vi "robotmovingFinal.vi"() -> ()   [LabVIEW 2020]
uses:
  <vilib>/Instr/_visa.llb/VISA Configure Serial Port (Instr).vi
panel:
  out "read buffer":string
  in  "VISA resource name":refnum<visa-resource-name>="COM3"
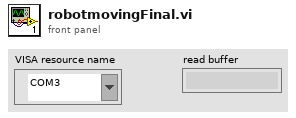
[diagram p1: front panel]
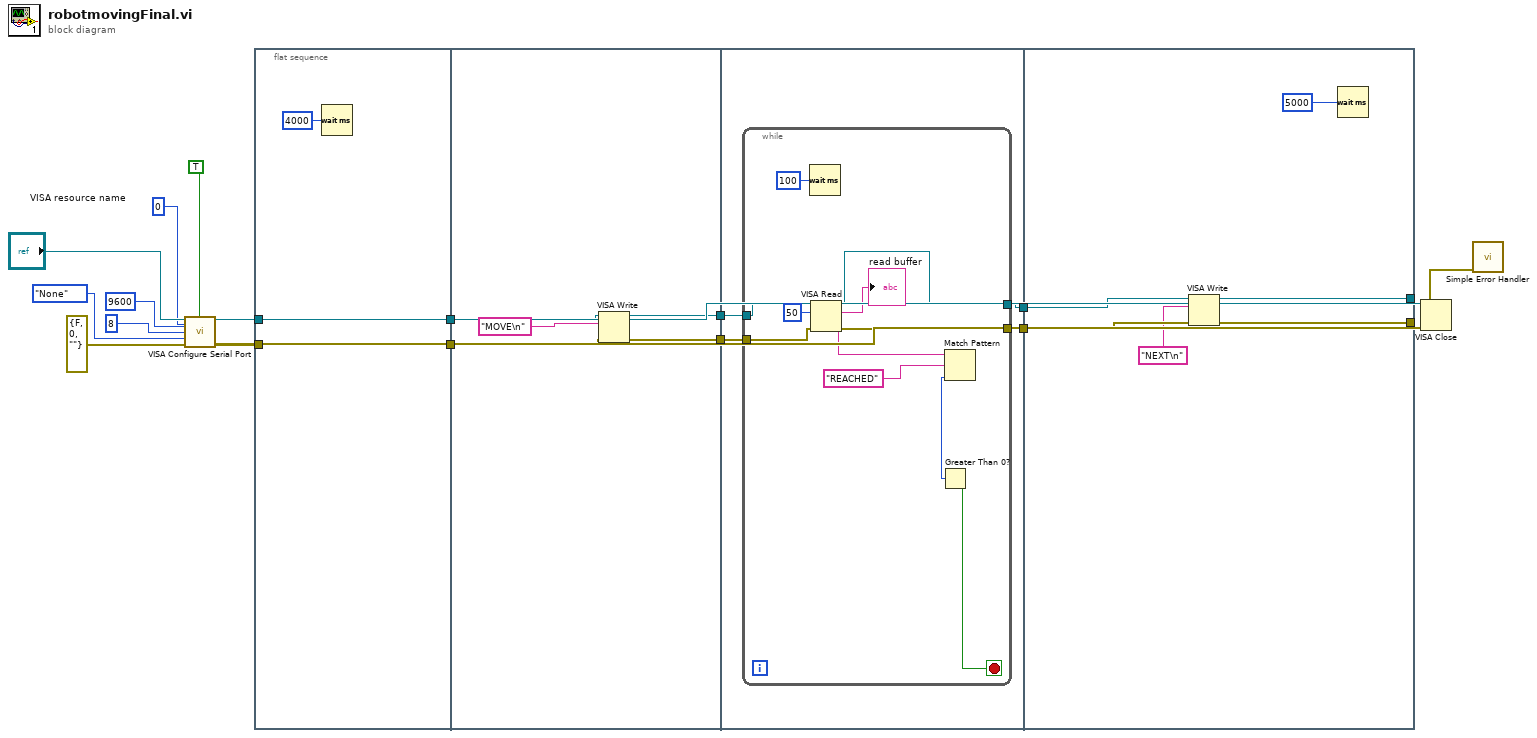
[diagram p0: block diagram]
diagram:
  n1 = call-poly "VISA Configure Serial Port"("VISA resource name"="VISA resource name", "termination char\n(0xA = '\\n' = LF)"=u8 0 ("termination char\n(0xA = '\\n' = LF)"), "Enable Termination\nChar (T)"=TRUE ("Enable Termination\nChar (T)"), "baud rate (9600)"=u32 9600, "data bits (8)"=u16 8, "parity (0:none)"=enum16{"None", "Odd", "Even", "Mark", "Space"}."None", "error in (no error)"=errorcluster {"status"=FALSE, "code"=0, "source"=""}) -> ("VISA resource name out"=w4:refnum<visa-resource-name>, "error out"=w3:errorcluster)  [unwired: 7 in]
  n2 = flat-sequence {
    tunnel: w3 -> [w18]
    tunnel: w4 -> [w19]
    tunnel: [w19] -> w2
    tunnel: [w18] -> w1
    tunnel: [w23] -> w9
    tunnel: [w22] -> w8
    tunnel: w2 -> [w21]
    tunnel: w1 -> [w20]
    tunnel: w9 -> [w28]
    tunnel: w8 -> [w27]
    tunnel: [w26] -> w7
    tunnel: [w25] -> w6
    tunnel: w7 -> [w43]
    tunnel: w6 -> [w42]
    tunnel: [w40] -> _
    tunnel: [w39] -> _
    frame #0 {
      n3 = Wait (ms)(milliseconds to wait=u32 4000) -> ()  [unwired: 1 out]
    }
    frame #1 {
      n4 = VISA Write(VISA resource name=w21, write buffer="MOVE\n", error in (no error)=w20) -> (VISA resource name out=w23:refnum<visa-resource-name>, error out=w22:errorcluster)  [unwired: 1 out]
    }
    frame #2 {
      n5 = while {
        tunnel: w28 -> [w38]
        tunnel: w27 -> [w37]
        tunnel: [w31] -> w26
        tunnel: [w30] -> w25
        stop <- w33 stop-if-true
        n6 = Wait (ms)(milliseconds to wait=u32 100) -> ()  [unwired: 1 out]
        n7 = VISA Read(VISA resource name=w38, byte count=u32 50, error in (no error)=w37) -> (VISA resource name out=w30:refnum<visa-resource-name>, read buffer=w35:string, error out=w31:errorcluster)  [unwired: 1 out]
        "read buffer" <- w35
        n8 = Match Pattern(string=w35, regular expression="REACHED") -> (offset past match=w29:i32)  [unwired: 1 in, 3 out]
        n9 = Greater Than 0?(x=w29) -> (x > 0?=w33:bool)
      }
    }
    frame #3 {
      n10 = VISA Write(VISA resource name=w42, write buffer="NEXT\n", error in (no error)=w43) -> (VISA resource name out=w40:refnum<visa-resource-name>, error out=w39:errorcluster)  [unwired: 1 out]
      n11 = Wait (ms)(milliseconds to wait=u32 5000 ("millisecond timer value")) -> ()  [unwired: 1 out]
    }
  }
  n12 = VISA Close(VISA resource name=w4, error in (no error)=w3) -> (error out=w5:errorcluster)
  n13 = call <vilib>:"Simple Error Handler.vi"("error in (no error)"=w5) -> ()  [unwired: 4 in, 5 out]
